vi "Get Sample Rate.vi"(8 "error in (no error)":errorcluster, 11 "DeviceRefnum":u64) -> (0 "error out":errorcluster, 2 "Sample Rate (Hz)":u32, 3 "DeviceRefnum Out":u64)   [LabVIEW 2016]
doc: "Get actual sample rate the device is configured to."
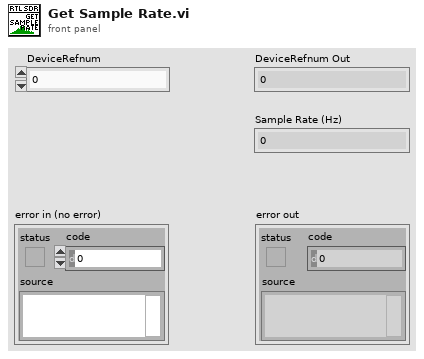
[diagram p1: front panel]
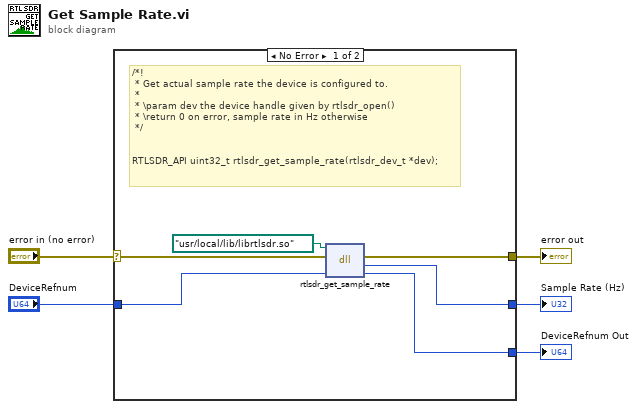
[diagram p0: block diagram]
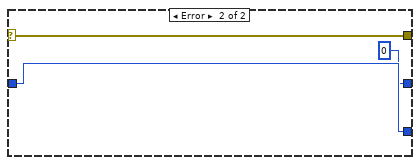
[diagram p2: hidden frame]
diagram:
  n1 = case shown="No Error" "error in (no error)" {
    selector: "error in (no error)" -> [w6 w14]
    tunnel: [w11 u32 0 ("return type")] -> w5
    tunnel: [w10 w14] -> w4
    tunnel: "DeviceRefnum" -> [w9 w13]
    tunnel: [w8 w13] -> w2
    frame No Error {
      # "/*!\n * Get actual sample rate the device is configured to.\n *\n * \\param dev the device handle given by rtlsdr_open()\n * \\return 0 on error, sample rate in Hz otherwise\n */\n\n\nRTLSDR_API uint32_t rtlsdr_get_sample_rate(rtlsdr_dev_t *dev);"
      n2 = dll-call lib="C:/Program Files (x86)/National Instruments/LabVIEW 2016/user.lib/rtlsdr/rtlsdr.*" fn="rtlsdr_get_sample_rate"(path in=path "/usr/local/lib/librtlsdr.so", error in=w6, "DeviceRefnum"=w9) -> (error out=w10:errorcluster, "return type"=w11:u32, "DeviceRefnum"=w8:u64)  [unwired: 1 in, 1 out]
    }
    frame Error {
    }
  }
  "Sample Rate (Hz)" <- w5
  "error out" <- w4
  "DeviceRefnum Out" <- w2
